vi "Version_4.9_8_on-chip_valves_for25ulSyringe_withModfied_Plunging.vi"() -> ()   [LabVIEW 2020] (continued)
                                }
                                }
                                n8038 = local write "Buffer-C Volume\nleft to be Pumped"(w8432) -> ()
                                }
                                frame #2 {
                                n8039 = local read "Buffer-C2 Dispense\nFlow Rate (ul/min)"() -> (w8459:dbl)
                                n8040 = local read "Buffer-C2 Pumping\nResolution"() -> (w8458:T2)
                                n8041 = local read "VISA Refnum in\nfor Pump"() -> (w8461:refnum<visa-resource-name>)
                                n8042 = local read "Volume of Syringe"() -> (w8460:dbl)
                                n8043 = call "GoToAbsolutePosition(SubVI).vi"("Absolute Volume Position in Syringe (in ul)"=0.0, "Volume of Syringe"=w8460, "Resolution of Pumping"=w8458, "Flow Rate (ul/min)"=w8459, "VISA Refnum in"=w8461) -> ()  [unwired: 6 in, 1 out]
                                n8044 = local write "Suction On/Off"(FALSE ("Suction On/Off")) -> ()
                                }
                                }
                                }
                                }
                                }
                                frame #4 {
                                n8045 = local read "Stop for End of \nExperiment \nand Data Writing"() -> (w8464:bool)
                                n8046 = local read "Re-SEC"() -> (w8463:bool)
                                n8047 = Or(x=w8464, y=w8463) -> (x .or. y?=w8462:bool)
                                n8048 = case shown="True" w8462 {
                                frame False {
                                }
                                frame True {
                                n8049 = local read "VISA Refnum in\nfor Pump"() -> (w8465:refnum<visa-resource-name>)
                                n8050 = call "HardStopCurrentProcess (SubVI).vi"("VISA Refnum in"=w8465) -> ()  [unwired: 11 in]
                                }
                                }
                                }
                                }
                              }
                              frame #2 {
                                # "Keeps the on-chip valve V1, V2 Open and V3 closed"
                                n8051 = while {
                                stop <- w8471 stop-if-true
                                n8052 = local read "Suction On/Off"() -> (w8472:bool)
                                n8053 = case shown="True" w8472 {
                                frame False {
                                n8054 = local read "Buffer-C2 Pumping\nResolution"() -> (w8478:T2)
                                n8055 = local read "Initial Plunger Position"() -> (w8477:dbl)
                                n8056 = local read "VISA Refnum in\nfor Pump"() -> (w8479:refnum<visa-resource-name>)
                                n8057 = local read "Position\nNow"() -> (w8475:dbl)
                                n8058 = local read "Volume of Syringe"() -> (w8476:dbl)
                                n8059 = local write "Volume being Injected \nin this process"(0.0) -> ()
                                n8060 = local write "Pause Data Collection"(FALSE) -> ()
                                n8061 = while {
                                tunnel: w8479 -> [w8486]
                                tunnel: w8478 -> [w8485]
                                tunnel: w8477 -> [w8481]
                                tunnel: w8476 -> [w8484]
                                tunnel: w8475 -> [w8480]
                                stop <- w8482 stop-if-true
                                n8062 = stacked-sequence {
                                tunnel: w8486 -> [w8492 w8514 w8541]
                                tunnel: w8485 -> [w8491 w8513 _]
                                tunnel: w8481 -> [w8489 _ _]
                                tunnel: w8484 -> [w8488 w8511 _]
                                tunnel: [_ _ w8534] -> w8482
                                tunnel: w8480 -> [_ w8509 _]
                                frame #0 {
                                # "From here on 'True Volume being injected \nin this process' represents the true total \nvolume in this process"
                                n8063 = call "AbsolutePlungerPosition (SubVI).vi"("VISA Refnum in"=w8492) -> ("Plunger Position"=w8490:i32)  [unwired: 10 in]
                                n8064 = case shown="..\"Standard Pumping\"" w8491 {
                                tunnel: w8490 -> [w8500 w8508]
                                tunnel: w8489 -> [w8499 w8507]
                                tunnel: w8488 -> [w8496 w8504]
                                tunnel: [w8493 w8501] -> w8487
                                frame .."Standard Pumping" {
                                n8065 = Subtract(x=w8500, y=w8499) -> (x-y=w8498:dbl)
                                n8066 = Absolute Value(x=w8498) -> (abs(x)=w8497:dbl)
                                n8067 = Multiply(x=w8497, y=w8496) -> (x*y=w8495:dbl)
                                n8068 = Divide(x=w8495, y=3000.0) -> (x/y=w8493:dbl)
                                }
                                frame "High Resolution Pumping".. {
                                n8069 = Subtract(x=w8508, y=w8507) -> (x-y=w8506:dbl)
                                n8070 = Absolute Value(x=w8506) -> (abs(x)=w8505:dbl)
                                n8071 = Multiply(x=w8505, y=w8504) -> (x*y=w8503:dbl)
                                n8072 = Divide(x=w8503, y=24000.0) -> (x/y=w8501:dbl)
                                }
                                }
                                n8073 = local write "True Volume being \ninjected in this\nprocess"(w8487) -> ()
                                }
                                frame #1 {
                                # "From here on 'Volume being injected \nin this process' represents the volume \nin this sub process"
                                n8074 = call "AbsolutePlungerPosition (SubVI).vi"("VISA Refnum in"=w8514) -> ("Plunger Position"=w8512:i32)  [unwired: 10 in]
                                n8075 = case shown="\"High Resolution Pumping\".." w8513 {
                                tunnel: w8512 -> [w8522 w8530]
                                tunnel: w8509 -> [w8521 w8529]
                                tunnel: w8511 -> [w8518 w8526]
                                tunnel: [w8515 w8523] -> w8510
                                frame .."Standard Pumping" {
                                n8076 = Subtract(x=w8522, y=w8521) -> (x-y=w8520:dbl)
                                n8077 = Absolute Value(x=w8520) -> (abs(x)=w8519:dbl)
                                n8078 = Multiply(x=w8519, y=w8518) -> (x*y=w8517:dbl)
                                n8079 = Divide(x=w8517, y=3000.0) -> (x/y=w8515:dbl)
                                }
                                frame "High Resolution Pumping".. {
                                n8080 = Subtract(x=w8530, y=w8529) -> (x-y=w8528:dbl)
                                n8081 = Absolute Value(x=w8528) -> (abs(x)=w8527:dbl)
                                n8082 = Multiply(x=w8527, y=w8526) -> (x*y=w8525:dbl)
                                n8083 = Divide(x=w8525, y=24000.0) -> (x/y=w8523:dbl)
                                }
                                }
                                n8084 = local write "Volume being Injected \nin this process"(w8510) -> ()
                                }
                                frame #2 {
                                n8085 = local read "Stop for End of \nExperiment \nand Data Writing"() -> (w8533:bool)
                                n8086 = local read "Re-SEC"() -> (w8532:bool)
                                n8087 = local read "Suction On/Off"() -> (w8537:bool)
                                n8088 = call "AbsolutePlungerPositionStatus (SubVI).vi"("VISA Refnum in"=w8541) -> ("read buffer"=w8540:string)  [unwired: 10 in]
                                n8089 = call <vilib>:"Trim Whitespace.vi"("string"=w8540) -> ("trimmed string"=w8539:string)  [unwired: 1 in]
                                n8090 = Equal?(x=w8539, y="/0`\u0003") -> (x = y?=w8536:bool)
                                n8091 = Or(x=w8533, y=w8532) -> (x .or. y?=w8531:bool)
                                n8092 = Or(x=w8537, y=w8531) -> (x .or. y?=w8535:bool)
                                n8093 = Or(x=w8536, y=w8535) -> (x .or. y?=w8534:bool)
                                }
                                }
                                n8094 = Wait (ms)(milliseconds to wait=u32 100) -> ()  [unwired: 1 out]
                                }
                                }
                                frame True {
                                n8095 = stacked-sequence {
                                frame #0 {
                                n8096 = local write "Valve V3 Open"(FALSE ("Valve V3 Open")) -> ()
                                n8097 = local read "Suction Pressure\nfor EM-grid \nDeposition (mbar)"() -> (w8548:sgl)
                                n8098 = local write "Valve V4 Open"(FALSE ("Valve V4 Open")) -> ()
                                n8099 = local read "VISA Refnum in\nfor Pump"() -> (w8551:refnum<visa-resource-name>)
                                n8100 = local write "Valve V5 Open"(FALSE ("Valve V1 Open")) -> ()
                                n8101 = local write "Suction pressure \nfor grid deposition"(w8548) -> ()
                                n8102 = local write "Re-deposit Sample\nonto Grid"(FALSE ("Redeposit Sample\nonto Grid")) -> ()
                                n8103 = local write "Pause Data Collection"(TRUE ("Pause Data Collection")) -> ()
                                n8104 = call "HardStopCurrentProcess (SubVI).vi"("VISA Refnum in"=w8551) -> ()  [unwired: 11 in]
                                n8105 = local write "Valve V6 Open"(TRUE ("Valve V2 Open")) -> ()
                                n8106 = local write "Valve V7 Open"(TRUE ("Valve V3 Open")) -> ()
                                n8107 = local write "External Valve \nOpen"(FALSE ("External Valve \nOpen")) -> ()
                                }
                                frame #1 {
                                n8108 = while {
                                stop <- w8554 stop-if-true
                                n8109 = local read "Stop for End of \nExperiment \nand Data Writing"() -> (w8555:bool)
                                n8110 = local read "Suction Pressure\nfor EM-grid \nDeposition (mbar)"() -> (w8552:sgl)
                                n8111 = call <vilib>:"fgt set pressure.vi"("pressure"=w8552, "pressureIndex"=u32 1) -> ()  [unwired: 9 in, 1 out]
                                n8112 = local read "Suction On/Off"() -> (w8557:bool)
                                n8113 = Not(x=w8557) -> (.not. x?=w8556:bool)
                                n8114 = Wait (ms)(milliseconds to wait=u32 100) -> ()  [unwired: 1 out]
                                n8115 = Or(x=w8556, y=w8555) -> (x .or. y?=w8554:bool)
                                }
                                }
                                frame #2 {
                                n8116 = for {
                                N: 2 -> [_]
                                n8117 = while {
                                stop <- w8567 stop-if-true
                                n8118 = local read "Stop for End of \nExperiment \nand Data Writing"() -> (w8563:bool)
                                n8119 = local read "Suction On/Off"() -> (w8565:bool)
                                n8120 = call <vilib>:"fgt set pressure.vi"("pressure"=sgl 0.0, "pressureIndex"=u32 1) -> ()  [unwired: 9 in, 1 out]
                                n8121 = Not(x=w8565) -> (.not. x?=w8564:bool)
                                n8122 = Wait (ms)(milliseconds to wait=u32 100) -> ()  [unwired: 1 out]
                                n8123 = Or(x=w8564, y=w8563) -> (x .or. y?=w8567:bool)
                                }
                                n8124 = Wait (ms)(milliseconds to wait=u32 400) -> ()  [unwired: 1 out]
                                }
                                }
                                frame #3 {
                                n8125 = local read "Automatic purging \nof capillary after \ngrid deposition"() -> (w8568:bool)
                                n8126 = case shown="True" w8568 {
                                frame False {
                                }
                                frame True {
                                n8127 = stacked-sequence {
                                frame #0 {
                                n8128 = local read "VISA Refnum in\nfor Pump"() -> (w8570:refnum<visa-resource-name>)
                                n8129 = call "AbsolutePlungerPosition (SubVI).vi"("VISA Refnum in"=w8570) -> ("Plunger Position"=w8569:i32)  [unwired: 10 in]
                                n8130 = local write "Position\nNow"(w8569) -> ()
                                }
                                frame #1 {
                                n8131 = local read "Buffer-C2 Pumping\nResolution"() -> (w8572:T2)
                                n8132 = case shown="\"Standard Pumping\", Default" w8572 {
                                tunnel: [w8573 w8584] -> w8571
                                frame "Standard Pumping", Default {
                                n8133 = local read "Buffer-C2 Volume \nto be Pumped"() -> (w8576:dbl)
                                n8134 = local read "Volume of Syringe"() -> (w8579:dbl)
                                n8135 = local read "Initial Plunger Position"() -> (w8583:dbl)
                                n8136 = local read "Position\nNow"() -> (w8582:dbl)
                                n8137 = Subtract(x=w8583, y=w8582) -> (x-y=w8581:dbl)
                                n8138 = Absolute Value(x=w8581) -> (abs(x)=w8580:dbl)
                                n8139 = Multiply(x=w8580, y=w8579) -> (x*y=w8578:dbl)
                                n8140 = Divide(x=w8578, y=3000.0) -> (x/y=w8575:dbl)
                                n8141 = Subtract(x=w8575, y=w8576) -> (x-y=w8574:dbl)
                                n8142 = Absolute Value(x=w8574) -> (abs(x)=w8573:dbl)
                                }
                                frame "High Resolution Pumping" {
                                n8143 = local read "Buffer-C2 Volume \nto be Pumped"() -> (w8587:dbl)
                                n8144 = local read "Volume of Syringe"() -> (w8590:dbl)
                                n8145 = local read "Initial Plunger Position"() -> (w8594:dbl)
                                n8146 = local read "Position\nNow"() -> (w8593:dbl)
                                n8147 = Subtract(x=w8594, y=w8593) -> (x-y=w8592:dbl)
                                n8148 = Absolute Value(x=w8592) -> (abs(x)=w8591:dbl)
                                n8149 = Multiply(x=w8591, y=w8590) -> (x*y=w8589:dbl)
                                n8150 = Divide(x=w8589, y=24000.0) -> (x/y=w8586:dbl)
                                n8151 = Subtract(x=w8586, y=w8587) -> (x-y=w8585:dbl)
                                n8152 = Absolute Value(x=w8585) -> (abs(x)=w8584:dbl)
                                }
                                }
                                n8153 = local write "Buffer-C Volume\nleft to be Pumped"(w8571) -> ()
                                }
                                frame #2 {
                                n8154 = local read "Buffer-C2 Dispense\nFlow Rate (ul/min)"() -> (w8603:dbl)
                                n8155 = local read "Buffer-C2 Pumping\nResolution"() -> (w8602:T2)
                                n8156 = local read "VISA Refnum in\nfor Pump"() -> (w8605:refnum<visa-resource-name>)
                                n8157 = local read "Volume of Syringe"() -> (w8604:dbl)
                                n8158 = call "GoToAbsolutePosition(SubVI).vi"("Absolute Volume Position in Syringe (in ul)"=0.0, "Volume of Syringe"=w8604, "Resolution of Pumping"=w8602, "Flow Rate (ul/min)"=w8603, "VISA Refnum in"=w8605) -> ()  [unwired: 6 in, 1 out]
                                n8159 = local write "External Valve \nOpen"(FALSE ("External Valve \nOpen")) -> ()
                                n8160 = local write "Valve V3 Open"(TRUE ("Valve V3 Open")) -> ()
                                n8161 = local write "Valve V7 Open"(FALSE ("Valve V3 Open")) -> ()
                                n8162 = local write "Valve V5 Open"(TRUE ("Valve V1 Open")) -> ()
                                n8163 = local write "Valve V6 Open"(TRUE ("Valve V2 Open")) -> ()
                                n8164 = local write "Valve V4 Open"(TRUE ("Valve V4 Open")) -> ()
                                }
                                frame #3 {
                                n8165 = local read "Buffer-C2 Pumping\nResolution"() -> (w8611:T2)
                                n8166 = local read "Initial Plunger Position"() -> (w8610:dbl)
                                n8167 = local read "VISA Refnum in\nfor Pump"() -> (w8612:refnum<visa-resource-name>)
                                n8168 = local read "Position\nNow"() -> (w8608:dbl)
                                n8169 = local read "Volume of Syringe"() -> (w8609:dbl)
                                n8170 = local write "Volume being Injected \nin this process"(0.0) -> ()
                                n8171 = local write "Pause Data Collection"(FALSE) -> ()
                                n8172 = while {
                                tunnel: w8612 -> [w8619]
                                tunnel: w8611 -> [w8618]
                                tunnel: w8610 -> [w8614]
                                tunnel: w8609 -> [w8617]
                                tunnel: w8608 -> [w8613]
                                stop <- w8615 stop-if-true
                                n8173 = stacked-sequence {
                                tunnel: w8619 -> [w8625 w8647 w8676]
                                tunnel: w8618 -> [w8624 w8646 _]
                                tunnel: w8614 -> [w8622 _ _]
                                tunnel: w8617 -> [w8621 w8644 _]
                                tunnel: [_ _ w8670] -> w8615
                                tunnel: w8613 -> [_ w8642 _]
                                frame #0 {
                                # "From here on 'True Volume being injected \nin this process' represents the true total \nvolume in this process"
                                n8174 = call "AbsolutePlungerPosition (SubVI).vi"("VISA Refnum in"=w8625) -> ("Plunger Position"=w8623:i32)  [unwired: 10 in]
                                n8175 = case shown="..\"Standard Pumping\"" w8624 {
                                tunnel: w8623 -> [w8633 w8641]
                                tunnel: w8622 -> [w8632 w8640]
                                tunnel: w8621 -> [w8629 w8637]
                                tunnel: [w8626 w8634] -> w8620
                                frame .."Standard Pumping" {
                                n8176 = Subtract(x=w8633, y=w8632) -> (x-y=w8631:dbl)
                                n8177 = Absolute Value(x=w8631) -> (abs(x)=w8630:dbl)
                                n8178 = Multiply(x=w8630, y=w8629) -> (x*y=w8628:dbl)
                                n8179 = Divide(x=w8628, y=3000.0) -> (x/y=w8626:dbl)
                                }
                                frame "High Resolution Pumping".. {
                                n8180 = Subtract(x=w8641, y=w8640) -> (x-y=w8639:dbl)
                                n8181 = Absolute Value(x=w8639) -> (abs(x)=w8638:dbl)
                                n8182 = Multiply(x=w8638, y=w8637) -> (x*y=w8636:dbl)
                                n8183 = Divide(x=w8636, y=24000.0) -> (x/y=w8634:dbl)
                                }
                                }
                                n8184 = local write "True Volume being \ninjected in this\nprocess"(w8620) -> ()
                                }
                                frame #1 {
                                # "From here on 'Volume being injected \nin this process' represents the volume \nin this sub process"
                                n8185 = call "AbsolutePlungerPosition (SubVI).vi"("VISA Refnum in"=w8647) -> ("Plunger Position"=w8645:i32)  [unwired: 10 in]
                                n8186 = case shown="\"High Resolution Pumping\".." w8646 {
                                tunnel: w8645 -> [w8655 w8663]
                                tunnel: w8642 -> [w8654 w8662]
                                tunnel: w8644 -> [w8651 w8659]
                                tunnel: [w8648 w8656] -> w8643
                                frame .."Standard Pumping" {
                                n8187 = Subtract(x=w8655, y=w8654) -> (x-y=w8653:dbl)
                                n8188 = Absolute Value(x=w8653) -> (abs(x)=w8652:dbl)
                                n8189 = Multiply(x=w8652, y=w8651) -> (x*y=w8650:dbl)
                                n8190 = Divide(x=w8650, y=3000.0) -> (x/y=w8648:dbl)
                                }
                                frame "High Resolution Pumping".. {
                                n8191 = Subtract(x=w8663, y=w8662) -> (x-y=w8661:dbl)
                                n8192 = Absolute Value(x=w8661) -> (abs(x)=w8660:dbl)
                                n8193 = Multiply(x=w8660, y=w8659) -> (x*y=w8658:dbl)
                                n8194 = Divide(x=w8658, y=24000.0) -> (x/y=w8656:dbl)
                                }
                                }
                                n8195 = local write "Volume being Injected \nin this process"(w8643) -> ()
                                }
                                frame #2 {
                                n8196 = local read "Capillary purge \nvolume after every\ngrid plunging"() -> (w8665:dbl)
                                n8197 = local read "Stop for End of \nExperiment \nand Data Writing"() -> (w8669:bool)
                                n8198 = local read "Volume being Injected \nin this process"() -> (w8666:dbl)
                                n8199 = local read "Re-SEC"() -> (w8668:bool)
                                n8200 = call "AbsolutePlungerPositionStatus (SubVI).vi"("VISA Refnum in"=w8676) -> ("read buffer"=w8675:string)  [unwired: 10 in]
                                n8201 = call <vilib>:"Trim Whitespace.vi"("string"=w8675) -> ("trimmed string"=w8674:string)  [unwired: 1 in]
                                n8202 = Greater Or Equal?(x=w8666, y=w8665) -> (x >= y?=w8664:bool)
                                n8203 = Equal?(x=w8674, y="/0`\u0003") -> (x = y?=w8672:bool)
                                n8204 = Or(x=w8669, y=w8668) -> (x .or. y?=w8667:bool)
                                n8205 = Or(x=w8664, y=w8667) -> (x .or. y?=w8671:bool)
                                n8206 = Or(x=w8672, y=w8671) -> (x .or. y?=w8670:bool)
                                }
                                }
                                n8207 = Wait (ms)(milliseconds to wait=u32 100) -> ()  [unwired: 1 out]
                                }
                                }
                                frame #4 {
                                n8208 = local read "VISA Refnum in\nfor Pump"() -> (w8677:refnum<visa-resource-name>)
                                n8209 = call "HardStopCurrentProcess (SubVI).vi"("VISA Refnum in"=w8677) -> ()  [unwired: 11 in]
                                }
                                }
                                }
                                }
                                }
                                frame #4 {
                                n8210 = local write "Valve V3 Open"(FALSE ("Valve V3 Open")) -> ()
                                n8211 = local write "Valve V7 Open"(FALSE ("Valve V3 Open")) -> ()
                                n8212 = local write "Valve V5 Open"(FALSE ("Valve V1 Open")) -> ()
                                n8213 = local write "Valve V6 Open"(FALSE ("Valve V2 Open")) -> ()
                                n8214 = local write "Valve V4 Open"(FALSE ("Valve V4 Open")) -> ()
                                }
                                frame #5 {
                                n8215 = while {
                                stop <- w8687 stop-if-true
                                n8216 = local read "Stop for End of \nExperiment \nand Data Writing"() -> (w8685:bool)
                                n8217 = local read "Re-deposit Sample\nonto Grid"() -> (w8688:bool)
                                n8218 = local read "Re-SEC"() -> (w8686:bool)
                                n8219 = Or(x=w8685, y=w8686) -> (x .or. y?=w8684:bool)
                                n8220 = Or(x=w8688, y=w8684) -> (x .or. y?=w8687:bool)
                                }
                                n8221 = One Button Dialog(message="Do you want to deposit sample on another grid? If yes, turn on 'Re-deposit Sample onto Grid'. Else turn on Re-SEC to do SEC again or STOP to end the experiment") -> ()  [unwired: 1 in, 1 out]
                                }
                                frame #6 {
                                n8222 = local write "Valve V4 Open"(TRUE ("Valve V4 Open")) -> ()
                                n8223 = local write "Valve V3 Open"(TRUE ("Valve V3 Open")) -> ()
                                n8224 = local write "Valve V7 Open"(FALSE ("Valve V3 Open")) -> ()
                                n8225 = local write "Valve V5 Open"(TRUE ("Valve V1 Open")) -> ()
                                n8226 = local write "Valve V6 Open"(TRUE ("Valve V2 Open")) -> ()
                                }
                                frame #7 {
                                n8227 = local read "Re-deposit Sample\nonto Grid"() -> (w8694:bool)
                                n8228 = case shown="True" w8694 {
                                frame False {
                                n8229 = local write "Suction On/Off"(FALSE ("Suction On/Off")) -> ()
                                }
                                frame True {
                                n8230 = stacked-sequence {
                                frame #0 {
                                n8231 = local read "VISA Refnum in\nfor Pump"() -> (w8697:refnum<visa-resource-name>)
                                n8232 = call "AbsolutePlungerPosition (SubVI).vi"("VISA Refnum in"=w8697) -> ("Plunger Position"=w8696:i32)  [unwired: 10 in]
                                n8233 = local write "Position\nNow"(w8696) -> ()
                                }
                                frame #1 {
                                n8234 = local read "Buffer-C2 Pumping\nResolution"() -> (w8699:T2)
                                n8235 = case shown="\"Standard Pumping\", Default" w8699 {
                                tunnel: [w8700 w8711] -> w8698
                                frame "Standard Pumping", Default {
                                n8236 = local read "Buffer-C2 Volume \nto be Pumped"() -> (w8703:dbl)
                                n8237 = local read "Volume of Syringe"() -> (w8706:dbl)
                                n8238 = local read "Initial Plunger Position"() -> (w8710:dbl)
                                n8239 = local read "Position\nNow"() -> (w8709:dbl)
                                n8240 = Subtract(x=w8710, y=w8709) -> (x-y=w8708:dbl)
                                n8241 = Absolute Value(x=w8708) -> (abs(x)=w8707:dbl)
                                n8242 = Multiply(x=w8707, y=w8706) -> (x*y=w8705:dbl)
                                n8243 = Divide(x=w8705, y=3000.0) -> (x/y=w8702:dbl)
                                n8244 = Subtract(x=w8702, y=w8703) -> (x-y=w8701:dbl)
                                n8245 = Absolute Value(x=w8701) -> (abs(x)=w8700:dbl)
                                }
                                frame "High Resolution Pumping" {
                                n8246 = local read "Buffer-C2 Volume \nto be Pumped"() -> (w8714:dbl)
                                n8247 = local read "Volume of Syringe"() -> (w8717:dbl)
                                n8248 = local read "Initial Plunger Position"() -> (w8721:dbl)
                                n8249 = local read "Position\nNow"() -> (w8720:dbl)
                                n8250 = Subtract(x=w8721, y=w8720) -> (x-y=w8719:dbl)
                                n8251 = Absolute Value(x=w8719) -> (abs(x)=w8718:dbl)
                                n8252 = Multiply(x=w8718, y=w8717) -> (x*y=w8716:dbl)
                                n8253 = Divide(x=w8716, y=24000.0) -> (x/y=w8713:dbl)
                                n8254 = Subtract(x=w8713, y=w8714) -> (x-y=w8712:dbl)
                                n8255 = Absolute Value(x=w8712) -> (abs(x)=w8711:dbl)
                                }
                                }
                                n8256 = local write "Buffer-C Volume\nleft to be Pumped"(w8698) -> ()
                                }
                                frame #2 {
                                n8257 = local read "Buffer-C2 Dispense\nFlow Rate (ul/min)"() -> (w8725:dbl)
                                n8258 = local read "Buffer-C2 Pumping\nResolution"() -> (w8724:T2)
                                n8259 = local read "VISA Refnum in\nfor Pump"() -> (w8727:refnum<visa-resource-name>)
                                n8260 = local read "Volume of Syringe"() -> (w8726:dbl)
                                n8261 = call "GoToAbsolutePosition(SubVI).vi"("Absolute Volume Position in Syringe (in ul)"=0.0, "Volume of Syringe"=w8726, "Resolution of Pumping"=w8724, "Flow Rate (ul/min)"=w8725, "VISA Refnum in"=w8727) -> ()  [unwired: 6 in, 1 out]
                                n8262 = local write "Suction On/Off"(FALSE ("Suction On/Off")) -> ()
                                }
                                }
                                }
                                }
                                }
                                frame #8 {
                                n8263 = local read "Stop for End of \nExperiment \nand Data Writing"() -> (w8729:bool)
                                n8264 = local read "Re-SEC"() -> (w8730:bool)
                                n8265 = Or(x=w8729, y=w8730) -> (x .or. y?=w8728:bool)
                                n8266 = case shown="True" w8728 {
                                frame False {
                                }
                                frame True {
                                n8267 = local read "VISA Refnum in\nfor Pump"() -> (w8731:refnum<visa-resource-name>)
                                n8268 = call "HardStopCurrentProcess (SubVI).vi"("VISA Refnum in"=w8731) -> ()  [unwired: 11 in]
                                }
                                }
                                }
                                }
                                }
                                }
                                n8269 = local read "Stop for End of \nExperiment \nand Data Writing"() -> (w8467:bool)
                                n8270 = local read "Divert Sample \nonto Grid"() -> (w8470:bool)
                                n8271 = local read "Re-SEC"() -> (w8468:bool)
                                n8272 = Not(x=w8470) -> (.not. x?=w8469:bool)
                                n8273 = Or(x=w8467, y=w8468) -> (x .or. y?=w8466:bool)
                                n8274 = Or(x=w8469, y=w8466) -> (x .or. y?=w8471:bool)
                                }
                              }
                            }
                            n8275 = local write "Discard fluid \nprior to 1st \ndeposition"(TRUE ("Discard fluid \nprior to 1st \ndeposition")) -> ()
                          }
                        }
                      }
                      frame #17 {
                        n8276 = local read "Stopper that ends \nthe main loops"() -> (w8733:bool)
                        n8277 = local read "Re-SEC"() -> (w8734:bool)
                        n8278 = Wait (ms)(milliseconds to wait=u32 500) -> ()  [unwired: 1 out]
                        n8279 = Or(x=w8733, y=w8734) -> (x .or. y?=w8732:bool)
                        n8280 = case shown="True" w8732 {
                          frame False {
                          }
                          frame True {
                            n8281 = local read "VISA Refnum in\nfor Pump"() -> (w8739:refnum<visa-resource-name>)
                            n8282 = call "HardStopCurrentProcess (SubVI).vi"("VISA Refnum in"=w8739) -> ()  [unwired: 11 in]
                          }
                        }
                        n8283 = local write "Divert Sample \nonto Grid"(FALSE ("Divert Sample \nonto Grid")) -> ()
                        n8284 = local write "Pause Data Collection"(TRUE ("Pause Data Collection")) -> ()
                        n8285 = local write "Start the Process"(FALSE ("Start the Process")) -> ()
                      }
                      frame #18 {
                        n8286 = local read "Stop for End of \nExperiment \nand Data Writing"() -> (w8746:bool)
                        n8287 = local read "Start the Process"() -> (w8745:bool)
                        n8288 = Or(x=w8745, y=w8746) -> (x .or. y?=w8744:bool)
                        n8289 = case shown="False" w8744 {
                          frame False {
                            n8290 = while {
                              stop <- w8752 stop-if-true
                              n8291 = local read "Stop for End of \nExperiment \nand Data Writing"() -> (w8754:bool)
                              n8292 = local read "Start the Process"() -> (w8753:bool)
                              n8293 = Or(x=w8753, y=w8754) -> (x .or. y?=w8752:bool)
                              n8294 = Wait (ms)(milliseconds to wait=u32 100) -> ()  [unwired: 1 out]
                            }
                            n8295 = One Button Dialog(message="Do you want to re-introduce sample into column-2 and elute? If yes, adjust the re-introduction volume into column-2 and elution parameters for column-2 and turn on the 'Start the Process' button . If no, turn on the 'Stop for End of Experiment and Data Writing'.") -> ()  [unwired: 1 in, 1 out]
                          }
                          frame True {
                            n8296 = local read "Stop for End of \nExperiment \nand Data Writing"() -> (w8755:bool)
                            n8297 = case shown="True" w8755 {
                              frame False {
                              }
                              frame True {
                                n8298 = local write "Valve V1 Open"(FALSE ("Valve V1 Open")) -> ()
                                n8299 = local write "Valve V2 Open"(FALSE ("Valve V2 Open")) -> ()
                                n8300 = local write "Valve V4 Open"(FALSE ("Valve V4 Open")) -> ()
                                n8301 = local write "Valve V3 Open"(FALSE ("Valve V3 Open")) -> ()
                                n8302 = local write "Valve V5 Open"(FALSE ("Valve V5 Open")) -> ()
                                n8303 = local write "Valve V6 Open"(FALSE ("Valve V6 Open")) -> ()
                                n8304 = local write "Valve V7 Open"(FALSE ("Valve V7 Open")) -> ()
                              }
                            }
                          }
                        }
                        n8305 = local write "Sample Volume Diverted\ninto Column-2"(0.0 ("Sample Volume Diverted\ninto Column-2")) -> ()
                        n8306 = local write "Buffer-C Volume\nleft to be Pumped"(0.0 ("Buffer-C Volume\nleft to be Pumped")) -> ()
                        n8307 = local write "Vol_previous"(0.0 ("Vol_previous")) -> ()
                        n8308 = local write "Vol_now"(0.0 ("Vol_now")) -> ()
                        n8309 = local write "Elution of Column-2"(FALSE ("Elution of Column-2")) -> ()
                        n8310 = local write "SEC On"(FALSE ("SEC On")) -> ()
                        n8311 = local write "Volume being Injected \nin this process"(0.0 ("Volume being Injected \nin this process")) -> ()
                      }
                    }
                  }
                }
              }
              frame True {
                n8312 = local write "Pause Data Collection"(FALSE ("Pause Data Collection")) -> ()
              }
            }
          }
        }
        n8313 = local read "Stop for End of \nExperiment \nand Data Writing"() -> (w524:bool)
        n8314 = local write "Stopper that ends \nthe main loops"(w524) -> ()
        n8315 = local read "Stopper that ends \nthe main loops"() -> (w525:bool)
      }
      n8316 = invoke class="KCubeInertialMotorControl" method="CreateDevice"(reference=w74, error in=w81) -> (reference out=w76:refnum<k24>, error out=w75:errorcluster)  [unwired: 1 in, 1 out]
      n8317 = property class="KCubeInertialMotorControl"(reference=w76, error in=w75) -> (reference out=w85:refnum<k24>, error out=w79:errorcluster, "Device"=w77:refnum<k24>)
      n8318 = while {
        tunnel: w77 -> [w111]
        tunnel: [w109] -> w78
        tunnel: w79 -> [w107]
        tunnel: [w106] -> w80
        stop <- w110 stop-if-true
        n8319 = invoke class="KCubeInertialMotor" method="IsSettingsInitialized"(reference=w111, error in=w107) -> (reference out=w109:refnum<k24>, error out=w106:errorcluster, "IsSettingsInitialized"=w110:bool)  [unwired: 1 in]
        n8320 = Wait (ms)(milliseconds to wait=u32 50) -> ()  [unwired: 1 out]
      }
      n8321 = Get Date/Time In Seconds() -> (seconds since 1Jan1904=w37:timestamp)
      n8322 = Get Date/Time In Seconds() -> (seconds since 1Jan1904=w34:timestamp)
      n8323 = Get Date/Time In Seconds() -> (seconds since 1Jan1904=w46:timestamp)
      n8324 = Get Date/Time In Seconds() -> (seconds since 1Jan1904=w43:timestamp)
      n8325 = Get Date/Time In Seconds() -> (seconds since 1Jan1904=w54:timestamp)
      n8326 = Get Date/Time In Seconds() -> (seconds since 1Jan1904=w51:timestamp)
      n8327 = Get Date/Time In Seconds() -> (seconds since 1Jan1904=w95:timestamp)
      n8328 = Get Date/Time In Seconds() -> (seconds since 1Jan1904=w91:timestamp)
      n8329 = Get Date/Time In Seconds() -> (seconds since 1Jan1904=w67:timestamp)
      n8330 = Bundle By Name("Y"=dbl[] [], "t0"=w34, "dt"=0.001) -> (w32:waveform(dbl))  [unwired: 1 in]
      n8331 = Bundle By Name("Y"=dbl[] [], "t0"=w37, "dt"=0.001) -> (w33:waveform(dbl))  [unwired: 1 in]
      n8332 = Bundle By Name("Y"=dbl[] [], "t0"=w43, "dt"=0.001) -> (w41:waveform(dbl))  [unwired: 1 in]
      n8333 = Bundle By Name("Y"=dbl[] [], "t0"=w46, "dt"=0.001) -> (w42:waveform(dbl))  [unwired: 1 in]
      n8334 = Bundle By Name("Y"=dbl[] [], "t0"=w51, "dt"=0.001) -> (w49:waveform(dbl))  [unwired: 1 in]
      n8335 = Bundle By Name("Y"=dbl[] [], "t0"=w54, "dt"=0.001) -> (w50:waveform(dbl))  [unwired: 1 in]
      n8336 = Bundle By Name("Y"=dbl[] [], "t0"=w91, "dt"=0.001) -> (w90:waveform(dbl))  [unwired: 1 in]
      n8337 = Bundle By Name("Y"=dbl[] [], "t0"=w95, "dt"=0.001) -> (w94:waveform(dbl))  [unwired: 1 in]
      n8338 = invoke class="KCubeInertialMotor" method="StartPolling"(reference=w78, error in=w80, "ms"=250) -> (reference out=w10:refnum<k24>, error out=w9:errorcluster)  [unwired: 1 in, 2 out]
      n8339 = Bundle By Name("Y"=dbl[] [], "t0"=w67, "dt"=0.1) -> (w72:waveform(dbl))  [unwired: 1 in]
      n8340 = while {
        shift-right: [w8791] -> w87
        shift-left: w94 -> [w8798]
        shift-right: [w8783] -> w88
        shift-left: w90 -> [w8784]
        shift-right: [w8778] -> _
        shift-left: w50 -> [w8779]
        shift-right: [w8776] -> _
        shift-left: w49 -> [w8777]
        shift-right: [w8773] -> _
        shift-left: w42 -> [w8775]
        shift-right: [w8772] -> _
        shift-left: w41 -> [w8774]
        shift-right: [w8767] -> _
        shift-left: w32 -> [w8769]
        shift-right: [w8768] -> _
        shift-left: w33 -> [w8770]
        stop <- w8786 stop-if-true
        # "Voltage applied in volts\nfor Opamps"
        # "Input Voltage Circuit  for the Amplifier"
        # "Amplified Signal in Volts"
        n8341 = local read "Stop for End of \nExperiment \nand Data Writing"() -> (w8782:bool)
        n8342 = local read "Volume being Injected \ntill the end of previous \nprocess"() -> (w8789:dbl)
        n8343 = local read "Pause Data Collection"() -> (w8788:bool)
        n8344 = local read "Affinity Elution \nis Approaching"() -> (w8771:bool)
        n8345 = local read "Affinity Elution On"() -> (w8764:bool)
        n8346 = local read "Volume being Injected \nin this process"() -> (w8790:dbl)
        n8347 = local read "SEC On"() -> (w8781:bool)
        n8348 = case shown="True" w8788 {
          frame False {
          }
          frame True {
            n8349 = local read "Volume being Injected \ntill the end of previous \nprocess"() -> (w8851:dbl)
            n8350 = while {
              stop <- w8853 continue-if-true
              n8351 = Wait (ms)(milliseconds to wait=u32 10) -> ()  [unwired: 1 out]
              n8352 = local read "Pause Data Collection"() -> (w8853:bool)
            }
            n8353 = local read "Volume being Injected \nin this process"() -> (w8849:dbl)
            n8354 = Add(x=w8849, y=w8851) -> (x+y=w8850:dbl)
            n8355 = local write "Volume being Injected \ntill the end of previous \nprocess"(w8850) -> ()
          }
        }
        n8356 = case shown="True" w8782 {
          frame False {
          }
          frame True {
            n8357 = stacked-sequence {
              frame #0 {
                n8358 = local write "Stopper that ends \nthe main loops"(TRUE) -> ()
                n8359 = local write "Start the Process"(TRUE) -> ()
                n8360 = local write "Pause Data Collection"(FALSE) -> ()
                n8361 = local write "Pause /Continue"(FALSE) -> ()
                n8362 = Wait (ms)(milliseconds to wait=250) -> ()  [unwired: 1 out]
              }
              frame #1 {
              }
            }
          }
        }
        n8363 = Add(x=w8789, y=w8790) -> (x+y=w8785:dbl)
        n8364 = call "Convert from Dynamic Data4"("Dynamic Data Type"=w8785) -> ("Waveform"=w8765:waveform(dbl))  [unwired: 3 in]
        n8365 = local write "Total Volume \nbeing Injected"(w8785) -> ()
        n8366 = call-poly <vilib>:"Append Waveforms.vi"("waveform B"=w8765, "waveform A"=w8784) -> ("waveform out"=w8783:waveform(dbl))  [unwired: 8 in, 1 out]
        n8367 = call "DAQ AO-0"("data"=-5) -> ()  [unwired: 17 in, 2 out]
        n8368 = call "Convert from Dynamic Data2"("Dynamic Data Type"=w8783) -> ("Array"=w8793:dbl[])  [unwired: 3 in]
        n8369 = local read "Stopper that ends \nthe main loops"() -> (w8786:bool)
        n8370 = call "DAQ Assistant"() -> ("data"=w8797:dynamicdata)  [unwired: 17 in, 2 out]
        n8371 = call "Convert from Dynamic Data"("Dynamic Data Type"=w8797) -> ("Waveform"=w8796:waveform(dbl))  [unwired: 3 in]
        n8372 = Multiply(x=-1, y=w8796) -> (x*y=w8766:waveform(dbl))
        n8373 = case shown="True" w8781 {
          tunnel: w8779 -> [w8834 w8841]
          tunnel: w8766 -> [_ w8840]
          tunnel: [w8833 w8839] -> w8778
          tunnel: w8777 -> [w8832 w8837]
          tunnel: [w8831 w8835] -> w8776
          tunnel: w8765 -> [_ w8836]
          frame False {
            n8374 = call-poly <vilib>:"Append Waveforms.vi"("waveform B"=waveform(dbl) {"t0"=timestamp(0 s since 1904-01-01), "dt"=1.0, "Y"=[]}, "waveform A"=w8832) -> ("waveform out"=w8831:waveform(dbl))  [unwired: 8 in, 1 out]
            n8375 = call-poly <vilib>:"Append Waveforms.vi"("waveform B"=waveform(dbl) {"t0"=timestamp(0 s since 1904-01-01), "dt"=1.0, "Y"=[]}, "waveform A"=w8834) -> ("waveform out"=w8833:waveform(dbl))  [unwired: 8 in, 1 out]
          }
          frame True {
            n8376 = call-poly <vilib>:"Append Waveforms.vi"("waveform B"=w8836, "waveform A"=w8837) -> ("waveform out"=w8835:waveform(dbl))  [unwired: 8 in, 1 out]
            n8377 = call "Convert from Dynamic Data6"("Dynamic Data Type"=w8835) -> ("Array"=w8842:dbl[])  [unwired: 3 in]
            n8378 = call-poly <vilib>:"Append Waveforms.vi"("waveform B"=w8840, "waveform A"=w8841) -> ("waveform out"=w8839:waveform(dbl))  [unwired: 8 in, 1 out]
            n8379 = call "Convert from Dynamic Data7"("Dynamic Data Type"=w8839) -> ("Array"=w8843:dbl[])  [unwired: 3 in]
            n8380 = Bundle("Array"=w8842, "Array"=w8843) -> (→"Amplified Signal with Fluid Volume for SEC":cluster{"Array":dbl[], "Array":dbl[]})  [unwired: 1 in]
          }
        }
        n8381 = case shown="True" w8771 {
          tunnel: w8775 -> [w8819 w8826]
          tunnel: w8766 -> [_ w8825]
          tunnel: [w8818 w8824] -> w8773
          tunnel: w8774 -> [w8817 w8822]
          tunnel: [w8816 w8820] -> w8772
          tunnel: w8765 -> [_ w8821]
          frame False {
            n8382 = call-poly <vilib>:"Append Waveforms.vi"("waveform B"=waveform(dbl) {"t0"=timestamp(0 s since 1904-01-01), "dt"=1.0, "Y"=[]}, "waveform A"=w8817) -> ("waveform out"=w8816:waveform(dbl))  [unwired: 8 in, 1 out]
            n8383 = call-poly <vilib>:"Append Waveforms.vi"("waveform B"=waveform(dbl) {"t0"=timestamp(0 s since 1904-01-01), "dt"=1.0, "Y"=[]}, "waveform A"=w8819) -> ("waveform out"=w8818:waveform(dbl))  [unwired: 8 in, 1 out]
          }
          frame True {
            n8384 = call-poly <vilib>:"Append Waveforms.vi"("waveform B"=w8821, "waveform A"=w8822) -> ("waveform out"=w8820:waveform(dbl))  [unwired: 8 in, 1 out]
            n8385 = call "Convert from Dynamic Data10"("Dynamic Data Type"=w8820) -> ("Array"=w8827:dbl[])  [unwired: 3 in]
            n8386 = call-poly <vilib>:"Append Waveforms.vi"("waveform B"=w8825, "waveform A"=w8826) -> ("waveform out"=w8824:waveform(dbl))  [unwired: 8 in, 1 out]
            n8387 = call "Convert from Dynamic Data11"("Dynamic Data Type"=w8824) -> ("Array"=w8828:dbl[])  [unwired: 3 in]
            n8388 = Bundle("Array"=w8827, "Array"=w8828) -> (→"Amplified Signal with Fluid Volume Near Affinity Elution":cluster{"Array":dbl[], "Array":dbl[]})  [unwired: 1 in]
          }
        }
        n8389 = case shown="True" w8764 {
          tunnel: w8770 -> [w8804 w8811]
          tunnel: w8766 -> [_ w8810]
          tunnel: [w8803 w8809] -> w8768
          tunnel: w8769 -> [w8802 w8807]
          tunnel: [w8801 w8806] -> w8767
          tunnel: w8765 -> [_ w8805]
          frame False {
            n8390 = call-poly <vilib>:"Append Waveforms.vi"("waveform B"=waveform(dbl) {"t0"=timestamp(0 s since 1904-01-01), "dt"=1.0, "Y"=[]}, "waveform A"=w8802) -> ("waveform out"=w8801:waveform(dbl))  [unwired: 8 in, 1 out]
            n8391 = call-poly <vilib>:"Append Waveforms.vi"("waveform B"=waveform(dbl) {"t0"=timestamp(0 s since 1904-01-01), "dt"=1.0, "Y"=[]}, "waveform A"=w8804) -> ("waveform out"=w8803:waveform(dbl))  [unwired: 8 in, 1 out]
          }
          frame True {
            n8392 = call-poly <vilib>:"Append Waveforms.vi"("waveform B"=w8805, "waveform A"=w8807) -> ("waveform out"=w8806:waveform(dbl))  [unwired: 8 in, 1 out]
            n8393 = call "Convert from Dynamic Data8"("Dynamic Data Type"=w8806) -> ("Array"=w8812:dbl[])  [unwired: 3 in]
            n8394 = call-poly <vilib>:"Append Waveforms.vi"("waveform B"=w8810, "waveform A"=w8811) -> ("waveform out"=w8809:waveform(dbl))  [unwired: 8 in, 1 out]
            n8395 = call "Convert from Dynamic Data9"("Dynamic Data Type"=w8809) -> ("Array"=w8813:dbl[])  [unwired: 3 in]
            n8396 = Bundle("Array"=w8812, "Array"=w8813) -> (→"Amplified Signal with Fluid Volume for Affinity Elution":cluster{"Array":dbl[], "Array":dbl[]})  [unwired: 1 in]
          }
        }
        n8397 = call-poly <vilib>:"Append Waveforms.vi"("waveform B"=w8766, "waveform A"=w8798) -> ("waveform out"=w8791:waveform(dbl))  [unwired: 8 in, 1 out]
        n8398 = call "Convert from Dynamic Data3"("Dynamic Data Type"=w8791) -> ("Array"=w8794:dbl[])  [unwired: 3 in]
        n8399 = Bundle("Array"=w8793, "Array"=w8794) -> (→"Amplified Signal with Fluid Volume":cluster{"Array":dbl[], "Array":dbl[]})  [unwired: 1 in]
        n8400 = Wait Until Next ms Multiple(millisecond multiple=u32 400) -> ()  [unwired: 1 out]
      }
      n8401 = call-poly "VISA Configure Serial Port"("VISA resource name"=refnum<visa-resource-name> "COM7", "timeout (10sec)"=u32 1000, "baud rate (9600)"=u32 9600) -> ("VISA resource name out"=w69:refnum<visa-resource-name>, "error out"=w68:errorcluster)  [unwired: 11 in]
      n8402 = call <vilib>:"fgt init.vi"() -> ("error out"=w28:errorcluster)  [unwired: 11 in]
      n8403 = call <vilib>:"fgt init.vi"() -> ("error out"=w18:errorcluster)  [unwired: 11 in]
      n8404 = call <vilib>:"fgt init.vi"() -> ("error out"=w12:errorcluster)  [unwired: 11 in]
      n8405 = call <vilib>:"fgt init.vi"() -> ("error out"=w14:errorcluster)  [unwired: 11 in]
      n8406 = call <vilib>:"fgt init.vi"() -> ("error out"=w20:errorcluster)  [unwired: 11 in]
      n8407 = call <vilib>:"fgt init.vi"() -> ("error out"=w16:errorcluster)  [unwired: 11 in]
      n8408 = call <vilib>:"fgt init.vi"() -> ("error out"=w22:errorcluster)  [unwired: 11 in]
      n8409 = call <vilib>:"fgt init.vi"() -> ("error out"=w26:errorcluster)  [unwired: 11 in]
      n8410 = call <vilib>:"fgt init.vi"() -> ("error out"=w24:errorcluster)  [unwired: 11 in]
      n8411 = while {
        tunnel: w28 -> [w475]
        tunnel: [w474] -> w27
        tunnel: w26 -> [w473]
        tunnel: [w472] -> w25
        tunnel: w24 -> [w471]
        tunnel: [w470] -> w23
        tunnel: w22 -> [w469]
        tunnel: [w468] -> w21
        tunnel: w20 -> [w467]
        tunnel: [w466] -> w19
        tunnel: w18 -> [w465]
        tunnel: [w464] -> w17
        tunnel: w16 -> [w463]
        tunnel: [w462] -> w15
        tunnel: w14 -> [w461]
        tunnel: [w460] -> w13
        tunnel: w12 -> [w459]
        tunnel: [w458] -> w11
        stop <- w485 stop-if-true
        # "- Controls the 7 on-chip Valves. \n- By default pressure is applied to close them\n- On-chip Valve opening pressure is applied same as the \nsuction pressure for grid deposition on all the valves"
        n8412 = local read "Valve V1 Open"() -> (w505:bool)
        n8413 = local read "Valve V2 Open"() -> (w491:bool)
        n8414 = local read "Valve V3 Open"() -> (w490:bool)
        n8415 = local read "Valve V4 Open"() -> (w489:bool)
        n8416 = local read "Valve V5 Open"() -> (w488:bool)
        n8417 = local read "Valve V6 Open"() -> (w487:bool)
        n8418 = local read "Valve V7 Open"() -> (w486:bool)
        n8419 = Wait (ms)(milliseconds to wait=u32 100) -> ()  [unwired: 1 out]
        n8420 = local read "Valve V8 Open"() -> (w480:bool)
        n8421 = local read "On-Chip Valve \nClosing\nPressure (mbar)"() -> (w483:dbl)
        n8422 = local read "Stopper that ends \nthe main loops"() -> (w485:bool)
        n8423 = case shown="True" w505 {
          tunnel: [1 0 ("position")] -> w504
          frame False {
          }
          frame True {
          }
        }
        n8424 = case shown="True" w491 {
          tunnel: [1 0 ("position")] -> w502
          frame False {
          }
          frame True {
          }
        }
        n8425 = case shown="True" w490 {
          tunnel: [1 0 ("position")] -> w501
          frame False {
          }
          frame True {
          }
        }
        n8426 = case shown="True" w489 {
          tunnel: [1 0 ("position")] -> w498
          frame False {
          }
          frame True {
          }
        }
        n8427 = case shown="True" w488 {
          tunnel: [1 0 ("position")] -> w496
          frame False {
          }
          frame True {
          }
        }
        n8428 = case shown="True" w487 {
          tunnel: [1 0 ("position")] -> w494
          frame False {
          }
          frame True {
          }
        }
        n8429 = call <vilib>:"fgt set pressure.vi"("error in (no error)"=w475, "pressure"=w483, "pressureIndex"=0 ("module")) -> ("error out"=w474:errorcluster)  [unwired: 8 in]
        n8430 = call <vilib>:"fgt get pressure.vi"("pressureIndex"=u32 1) -> ("pressure out"=w478:sgl)  [unwired: 9 in, 1 out]
        n8431 = call <vilib>:"fgt get pressure.vi"("pressureIndex"=u32 0) -> ("pressure out"=w476:sgl)  [unwired: 9 in, 1 out]
        n8432 = case shown="True" w486 {
          tunnel: [1 0 ("position")] -> w492
          frame False {
          }
          frame True {
          }
        }
        n8433 = case shown="True" w480 {
          tunnel: [1 0 ("position")] -> w481
          frame False {
          }
          frame True {
          }
        }
        n8434 = call <vilib>:"fgt set valve position.vi"("error in (no error)"=w459, "position"=w504, "valveIndex"=u32 0) -> ("error out"=w458:errorcluster)  [unwired: 8 in]
        n8435 = call <vilib>:"fgt set valve position.vi"("error in (no error)"=w461, "position"=w502, "valveIndex"=u32 1) -> ("error out"=w460:errorcluster)  [unwired: 8 in]
        n8436 = call <vilib>:"fgt set valve position.vi"("error in (no error)"=w463, "position"=w501, "valveIndex"=u32 2) -> ("error out"=w462:errorcluster)  [unwired: 8 in]
        n8437 = call <vilib>:"fgt set valve position.vi"("error in (no error)"=w465, "position"=w498, "valveIndex"=u32 3) -> ("error out"=w464:errorcluster)  [unwired: 8 in]
        n8438 = call <vilib>:"fgt set valve position.vi"("error in (no error)"=w467, "position"=w496, "valveIndex"=u32 4) -> ("error out"=w466:errorcluster)  [unwired: 8 in]
        n8439 = call <vilib>:"fgt set valve position.vi"("error in (no error)"=w469, "position"=w494, "valveIndex"=u32 5) -> ("error out"=w468:errorcluster)  [unwired: 8 in]
        n8440 = local write "Valve Closing \nPressure Measured"(w476) -> ()
        n8441 = call <vilib>:"fgt set valve position.vi"("error in (no error)"=w471, "position"=w492, "valveIndex"=u32 6) -> ("error out"=w470:errorcluster)  [unwired: 8 in]
        n8442 = call <vilib>:"fgt set valve position.vi"("error in (no error)"=w473, "position"=w481, "valveIndex"=u32 7) -> ("error out"=w472:errorcluster)  [unwired: 8 in]
        n8443 = local write "Suction pressure \nmeasured"(w478) -> ()
      }
      n8444 = call <vilib>:"fgt close.vi"("error in (no error)"=w27) -> ()  [unwired: 10 in, 1 out]
      n8445 = call <vilib>:"fgt close.vi"("error in (no error)"=w17) -> ()  [unwired: 10 in, 1 out]
      n8446 = call <vilib>:"fgt close.vi"("error in (no error)"=w11) -> ()  [unwired: 10 in, 1 out]
      n8447 = call <vilib>:"fgt close.vi"("error in (no error)"=w13) -> ()  [unwired: 10 in, 1 out]
      n8448 = call <vilib>:"fgt close.vi"("error in (no error)"=w19) -> ()  [unwired: 10 in, 1 out]
      n8449 = call <vilib>:"fgt close.vi"("error in (no error)"=w15) -> ()  [unwired: 10 in, 1 out]
      n8450 = call <vilib>:"fgt close.vi"("error in (no error)"=w21) -> ()  [unwired: 10 in, 1 out]
      n8451 = call <vilib>:"fgt close.vi"("error in (no error)"=w25) -> ()  [unwired: 10 in, 1 out]
      n8452 = call <vilib>:"fgt close.vi"("error in (no error)"=w23) -> ()  [unwired: 10 in, 1 out]
      n8453 = while {
        stop <- w98 stop-if-true
        n8454 = event shown="[2] \"Stop for End of  Experiment  and Data Writing\": Value Change" {
          selector: _ -> [_ _ _]
          dyn-events: _ -> [_ _ _]
          timeout: 100 -> [_ _ _]
          tunnel: [_ _ w105] -> w98
          event Timeout {
            n8455 = event-data() -> ()  [unwired: 1 in, 3 out]
          }
          event "External Valve \nOpen": Value Change {
            n8456 = event-data() -> ()  [unwired: 1 in, 6 out]
            n8457 = local read "External Valve \nOpen"() -> (w100:bool)
            n8458 = case shown="False" w100 {
              frame False {
                # "external vale is closed"
                n8459 = local read "VISA Refnum in\nfor Valve"() -> (w102:refnum<visa-resource-name>)
                n8460 = call "PortChanger_Valve (SubVI).vi"("Port Number"="2", "VISA Refnum in"=w102) -> ()  [unwired: 10 in]
              }
              frame True {
                # "External valve is open"
                n8461 = local read "VISA Refnum in\nfor Valve"() -> (w104:refnum<visa-resource-name>)
                n8462 = call "PortChanger_Valve (SubVI).vi"("Port Number"="1", "VISA Refnum in"=w104) -> ()  [unwired: 10 in]
              }
            }
          }
          event "Stop for End of \nExperiment \nand Data Writing": Value Change {
            n8463 = event-data() -> ()  [unwired: 1 in, 6 out]
            n8464 = local read "Stop for End of \nExperiment \nand Data Writing"() -> (w105:bool)
          }
        }
      }
      n8465 = while {
        tunnel: [w120] -> w71
        tunnel: [w122] -> w70
        tunnel: w69 -> [w133]
        tunnel: w68 -> [w132]
        shift-right: [w121] -> _
        shift-left: w72 -> [w131]
        tunnel: [w130] -> w83
        tunnel: [w129] -> w84
        tunnel: w85 -> [w114]
        tunnel: [w114] -> w86
        tunnel: w10 -> [w112]
        tunnel: w9 -> [w113]
        stop <- w115 stop-if-true
        n8466 = local write "Position"(0 ("Position")) -> ()
        n8467 = local write "k1"(0.0 ("k1")) -> ()
        n8468 = local write "k2"(0.0 ("k2")) -> ()
        n8469 = event shown="[0] \"Select the Action\": Value Change" {
          selector: _ -> [_ _ _ _ _ _ _ _ _ _]
          dyn-events: _ -> [_ _ _ _ _ _ _ _ _ _]
          timeout: 100 -> [_ _ _ _ _ _ _ _ _ _]
          tunnel: w133 -> [w160 w407 w417 w428 w431 w436 w441 w446 w450 w457]
          tunnel: w132 -> [w159 w406 w416 w427 w432 w437 w442 w447 w449 w456]
          tunnel: w131 -> [_ _ _ _ _ _ _ _ _ _]
          tunnel: w112 -> [_ _ _ _ _ _ _ _ w452 w455]
          tunnel: w113 -> [_ _ _ _ _ _ _ _ w451 w454]
          tunnel: [w156 w404 w414 w424 _ _ _ _ w451 w454] -> w130
          tunnel: [w155 _ _ _ _ _ _ _ w452 w455] -> w129
          tunnel: [_ _ _ _ _ _ _ _ w453 _] -> w115
          tunnel: [w158 w405 w415 w425 w429 w434 w439 w444 w450 w457] -> w124
          tunnel: [w157 _ _ _ w430 w435 w440 w445 w449 w456] -> w123
          tunnel: w112 -> [w152 _ _ _ _ _ _ _ _ _]
          tunnel: w113 -> [w153 _ _ _ _ _ _ _ _ _]
          event "Select the Action": Value Change {
            n8470 = event-data() -> ()  [unwired: 1 in, 6 out]
            n8471 = local read "Select the Action"() -> (w154:T1)
            n8472 = case shown="\"Spread the deposited protein on the grid in One Line and plunge\"" w154 {
              tunnel: [w167 w174 w182 w266 w289 w377] -> w158
              tunnel: [w166 w173 w181 w265 w288 w376] -> w157
              tunnel: w160 -> [w165 w172 w180 w270 w287 w375]
              tunnel: w159 -> [w164 w171 w179 w269 w286 w374]
              tunnel: w152 -> [w161 w168 w178 w267 w285 w373]
              tunnel: w153 -> [w162 w169 w177 w268 w284 w372]
              tunnel: [w162 w169 w175 w268 w282 w372] -> w156
              tunnel: [w161 w168 w176 w267 w283 w373] -> w155
              frame .."Turn off Stepper Motor" {
                n8473 = VISA Write(VISA resource name=w165, write buffer="f", error in (no error)=w164) -> (VISA resource name out=w167:refnum<visa-resource-name>, error out=w166:errorcluster)  [unwired: 1 out]
              }
              frame "Turn  on Stepper Motor" {
                n8474 = VISA Write(VISA resource name=w172, write buffer="n", error in (no error)=w171) -> (VISA resource name out=w174:refnum<visa-resource-name>, error out=w173:errorcluster)  [unwired: 1 out]
              }
              frame "Start Plunging" {
                n8475 = stacked-sequence {
                  seq-local: [_ _ _ _ _ w204 _] -> [_ _ _ _ _ _ w263]
                  seq-local: [_ _ _ _ _ w203 _] -> [_ _ _ _ _ _ w262]
                  seq-local: [w184 _ _ _ _ _ _] -> [_ w191 _ _ _ _ _]
                  seq-local: [w183 _ _ _ _ _ _] -> [_ w190 _ _ _ _ _]
                  seq-local: [_ w189 _ _ _ _ _] -> [_ _ _ _ _ w202 _]
                  seq-local: [_ w188 _ _ _ _ _] -> [_ _ _ _ _ w201 _]
                  tunnel: [_ _ _ _ _ _ w261] -> w182
                  tunnel: [_ _ _ _ _ _ w260] -> w181
                  tunnel: w180 -> [_ _ _ _ _ w206 _]
                  tunnel: w179 -> [_ _ _ _ _ w205 _]
                  tunnel: w178 -> [w185 _ _ _ _ _ _]
                  tunnel: w177 -> [w186 _ _ _ _ _ _]
                  tunnel: [_ _ _ _ _ w200 _] -> w176
                  tunnel: [_ _ _ _ _ w199 _] -> w175
                  frame #0 {
                    w187 = 1 items=["Channel1"=1, "Channel2"=2, "Channel3"=3, "Channel4"=4] ("channel")
                    n8476 = invoke class="KCubeInertialMotor" method="SetPositionToZero"(reference=w185, error in=w186, "channel"=w187) -> (reference out=w184:refnum<k24>, error out=w183:errorcluster)  [unwired: 1 in, 2 out]
                  }
                  frame #1 {
                    w192 = 2 items=["Channel1"=1, "Channel2"=2, "Channel3"=3, "Channel4"=4] ("channel")
                    n8477 = invoke class="KCubeInertialMotor" method="SetPositionToZero"(reference=w191, error in=w190, "channel"=w192) -> (reference out=w189:refnum<k24>, error out=w188:errorcluster)  [unwired: 1 in, 2 out]
                  }
                  frame #2 {
                    n8478 = local write "Re-deposit Sample\nonto Grid"(FALSE ("Re-deposit Sample\nonto Grid")) -> ()
                    n8479 = local write "Divert Sample \nonto Grid"(TRUE ("Divert Sample \nonto Grid")) -> ()
                    n8480 = local read "Grid Deposition\nDuration"() -> (w193:u32)
                    n8481 = Wait (ms)(milliseconds to wait=w193) -> ()  [unwired: 1 out]
                  }
                  frame #3 {
                    n8482 = local write "Suction On/Off"(TRUE ("Suction On/Off")) -> ()
                  }
                  frame #4 {
                    n8483 = local read "Delay before\n1st movement\nof grid"() -> (w197:dbl)
                    n8484 = Wait (ms)(milliseconds to wait=w197) -> ()  [unwired: 1 out]
                  }
                  frame #5 {
                    n8485 = local read "No of cycles\nof up-down\nmovement"() -> (w198:dbl)
                    n8486 = for {
                      N: w198 -> [_]
                      shift-right: [w212] -> w204
                      shift-left: w206 -> [w214]
                      shift-right: [w211] -> w203
                      shift-left: w205 -> [w213]
                      shift-right: [w208] -> w200
                      shift-left: w202 -> [w210]
                      shift-right: [w207] -> w199
                      shift-left: w201 -> [w209]
                      n8487 = stacked-sequence {
                        seq-local: [w216 _ _ _ _ _] -> [_ _ _ w238 _ _]
                        seq-local: [w215 _ _ _ _ _] -> [_ _ _ w237 _ _]
                        seq-local: [_ _ w222 _ _ _] -> [_ _ _ _ _ w246]
                        seq-local: [_ _ w221 _ _ _] -> [_ _ _ _ _ w245]
                        tunnel: [_ _ _ w239 _ _] -> w212
                        tunnel: [_ _ _ w241 _ _] -> w211
                        tunnel: w214 -> [w219 _ _ _ _ _]
                        tunnel: w213 -> [w218 _ _ _ _ _]
                        tunnel: w210 -> [_ _ w224 _ _ _]
                        tunnel: w209 -> [_ _ w223 _ _ _]
                        tunnel: [_ _ _ _ _ w244] -> w208
                        tunnel: [_ _ _ _ _ w243] -> w207
                        frame #0 {
                          n8488 = VISA Write(VISA resource name=w219, write buffer="d", error in (no error)=w218) -> (VISA resource name out=w216:refnum<visa-resource-name>, error out=w215:errorcluster)  [unwired: 1 out]
                        }
                        frame #1 {
                          n8489 = local read "Duration for \nup/down\nMovement of Grid"() -> (w220:u32)
                          n8490 = Wait (ms)(milliseconds to wait=w220) -> ()  [unwired: 1 out]
                        }
                        frame #2 {
                          n8491 = stacked-sequence {
                            tunnel: w224 -> [_ w232 _]
                            tunnel: w223 -> [_ w231 _]
                            tunnel: [_ w230 _] -> w222
                            tunnel: [_ w229 _] -> w221
                            frame #0 {
                              n8492 = local read "Translation Step SIze\nwhile plunging"() -> (w225:dbl)
                              n8493 = local read "k1"() -> (w227:dbl)
                              n8494 = Decrement(x=w227) -> (x-1=w226:dbl)
                              n8495 = Multiply(x=w225, y=w226) -> (x*y=w228:dbl)
                              n8496 = local write "k2"(w226) -> ()
                              n8497 = local write "Position"(w228) -> ()
                            }
                            frame #1 {
                              w235 = 1 items=["Channel1"=1, "Channel2"=2, "Channel3"=3, "Channel4"=4] ("channel")
                              n8498 = local read "Position"() -> (w234:i32)
                              n8499 = invoke class="KCubeInertialMotor" method="MoveTo"(reference=w232, error in=w231, "channel"=w235, "position"=w234, "waitTimeout"=10000) -> (reference out=w230:refnum<k24>, error out=w229:errorcluster)  [unwired: 1 in, 4 out]
                            }
                            frame #2 {
                              n8500 = local read "Wait time for\ntranslation"() -> (w236:u32)
                              n8501 = Wait (ms)(milliseconds to wait=w236) -> ()  [unwired: 1 out]
                            }
                          }
                        }
                        frame #3 {
                          n8502 = VISA Write(VISA resource name=w238, write buffer="u", error in (no error)=w237) -> (VISA resource name out=w239:refnum<visa-resource-name>, error out=w241:errorcluster)  [unwired: 1 out]
                        }
                        frame #4 {
                          n8503 = local read "Duration for \nup/down\nMovement of Grid"() -> (w242:u32)
                          n8504 = Wait (ms)(milliseconds to wait=w242) -> ()  [unwired: 1 out]
                        }
                        frame #5 {
                          n8505 = stacked-sequence {
                            tunnel: w246 -> [_ w254 _]
                            tunnel: w245 -> [_ w253 _]
                            tunnel: [_ w252 _] -> w244
                            tunnel: [_ w251 _] -> w243
                            frame #0 {
                              n8506 = local read "Translation Step SIze\nwhile plunging"() -> (w247:dbl)
                              n8507 = local read "k2"() -> (w249:dbl)
                              n8508 = Increment(x=w249) -> (x+1=w248:dbl)
                              n8509 = Multiply(x=w247, y=w248) -> (x*y=w250:dbl)
                              n8510 = local write "k1"(w248) -> ()
                              n8511 = local write "Position"(w250) -> ()
                            }
                            frame #1 {
                              w257 = 1 items=["Channel1"=1, "Channel2"=2, "Channel3"=3, "Channel4"=4] ("channel")
                              n8512 = local read "Position"() -> (w256:i32)
                              n8513 = invoke class="KCubeInertialMotor" method="MoveTo"(reference=w254, error in=w253, "channel"=w257, "position"=w256, "waitTimeout"=10000) -> (reference out=w252:refnum<k24>, error out=w251:errorcluster)  [unwired: 1 in, 4 out]
                            }
                            frame #2 {
                              n8514 = local read "Wait time for\ntranslation"() -> (w258:u32)
                              n8515 = Wait (ms)(milliseconds to wait=w258) -> ()  [unwired: 1 out]
                            }
                          }
                        }
                      }
                    }
                  }
                  frame #6 {
                    n8516 = VISA Write(VISA resource name=w263, write buffer="p", error in (no error)=w262) -> (VISA resource name out=w261:refnum<visa-resource-name>, error out=w260:errorcluster)  [unwired: 1 out]
                    n8517 = local write "Suction On/Off"(FALSE ("Suction On/Off")) -> ()
                  }
                }
              }
              frame "Reset Plunger" {
                n8518 = stacked-sequence {
                  seq-local: [w272 _] -> [_ w280]
                  seq-local: [w271 _] -> [_ w279]
                  tunnel: w270 -> [w276 _]
                  tunnel: w269 -> [w275 _]
                  tunnel: [_ w278] -> w266
                  tunnel: [_ w277] -> w265
                  frame #0 {
                    n8519 = VISA Write(VISA resource name=w276, write buffer="r", error in (no error)=w275) -> (VISA resource name out=w272:refnum<visa-resource-name>, error out=w271:errorcluster)  [unwired: 1 out]
                    n8520 = Wait (ms)(milliseconds to wait=u32 1000) -> ()  [unwired: 1 out]
                  }
                  frame #1 {
                    n8521 = VISA Write(VISA resource name=w280, write buffer="f", error in (no error)=w279) -> (VISA resource name out=w278:refnum<visa-resource-name>, error out=w277:errorcluster)  [unwired: 1 out]
                  }
                }
              }
              frame "Spread the deposited protein on the grid and plunge" {
                n8522 = stacked-sequence {
                  seq-local: [_ _ _ _ _ w311 _] -> [_ _ _ _ _ _ w370]
                  seq-local: [_ _ _ _ _ w310 _] -> [_ _ _ _ _ _ w369]
                  seq-local: [w291 _ _ _ _ _ _] -> [_ w298 _ _ _ _ _]
                  seq-local: [w290 _ _ _ _ _ _] -> [_ w297 _ _ _ _ _]
                  seq-local: [_ w296 _ _ _ _ _] -> [_ _ _ _ _ w309 _]
                  seq-local: [_ w295 _ _ _ _ _] -> [_ _ _ _ _ w308 _]
                  tunnel: [_ _ _ _ _ _ w368] -> w289
                  tunnel: [_ _ _ _ _ _ w367] -> w288
                  tunnel: w287 -> [_ _ _ _ _ w313 _]
                  tunnel: w286 -> [_ _ _ _ _ w312 _]
                  tunnel: w285 -> [w292 _ _ _ _ _ _]
                  tunnel: w284 -> [w293 _ _ _ _ _ _]
                  tunnel: [_ _ _ _ _ w307 _] -> w283
                  tunnel: [_ _ _ _ _ w306 _] -> w282
                  frame #0 {
                    w294 = 1 items=["Channel1"=1, "Channel2"=2, "Channel3"=3, "Channel4"=4] ("channel")
                    n8523 = invoke class="KCubeInertialMotor" method="SetPositionToZero"(reference=w292, error in=w293, "channel"=w294) -> (reference out=w291:refnum<k24>, error out=w290:errorcluster)  [unwired: 1 in, 2 out]
                  }
                  frame #1 {
                    w299 = 2 items=["Channel1"=1, "Channel2"=2, "Channel3"=3, "Channel4"=4] ("channel")
                    n8524 = invoke class="KCubeInertialMotor" method="SetPositionToZero"(reference=w298, error in=w297, "channel"=w299) -> (reference out=w296:refnum<k24>, error out=w295:errorcluster)  [unwired: 1 in, 2 out]
                  }
                  frame #2 {
                    n8525 = local write "Re-deposit Sample\nonto Grid"(FALSE ("Re-deposit Sample\nonto Grid")) -> ()
                    n8526 = local write "Divert Sample \nonto Grid"(TRUE ("Divert Sample \nonto Grid")) -> ()
                    n8527 = local read "Grid Deposition\nDuration"() -> (w300:u32)
